vi "Update Methods Event Unbundlers.vi"(8 "error in (no error)":errorcluster, 10 "RPC Method Parameters":T1, 11 "LVClassLibrary in":refnum<vi>) -> (0 "error out":errorcluster, 3 "LVClassLibrary out":refnum<vi>)   [LabVIEW 2019, in "gRPC Template Creation Utility.lvlib"]
uses:
  gRPC Template Creation Utility.lvlib
  TypeDefs/RPC Method Parameters.ctl
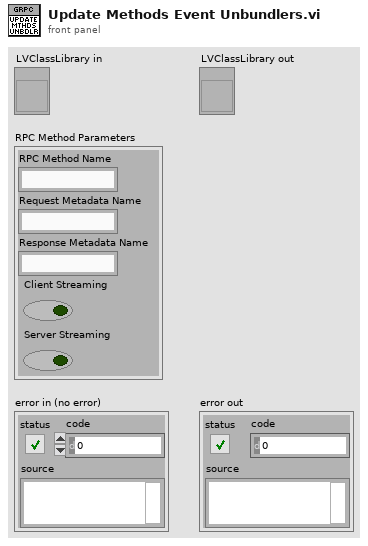
[diagram p1: front panel]
types:
  T1 = typedef "gRPC Template Creation Utility.lvlib/RPC Method Parameters.ctl" = cluster{"RPC Method Name":string, "Request Metadata Name":string, "Response Metadata Name":string, "Client Streaming":bool, "Server Streaming":bool}
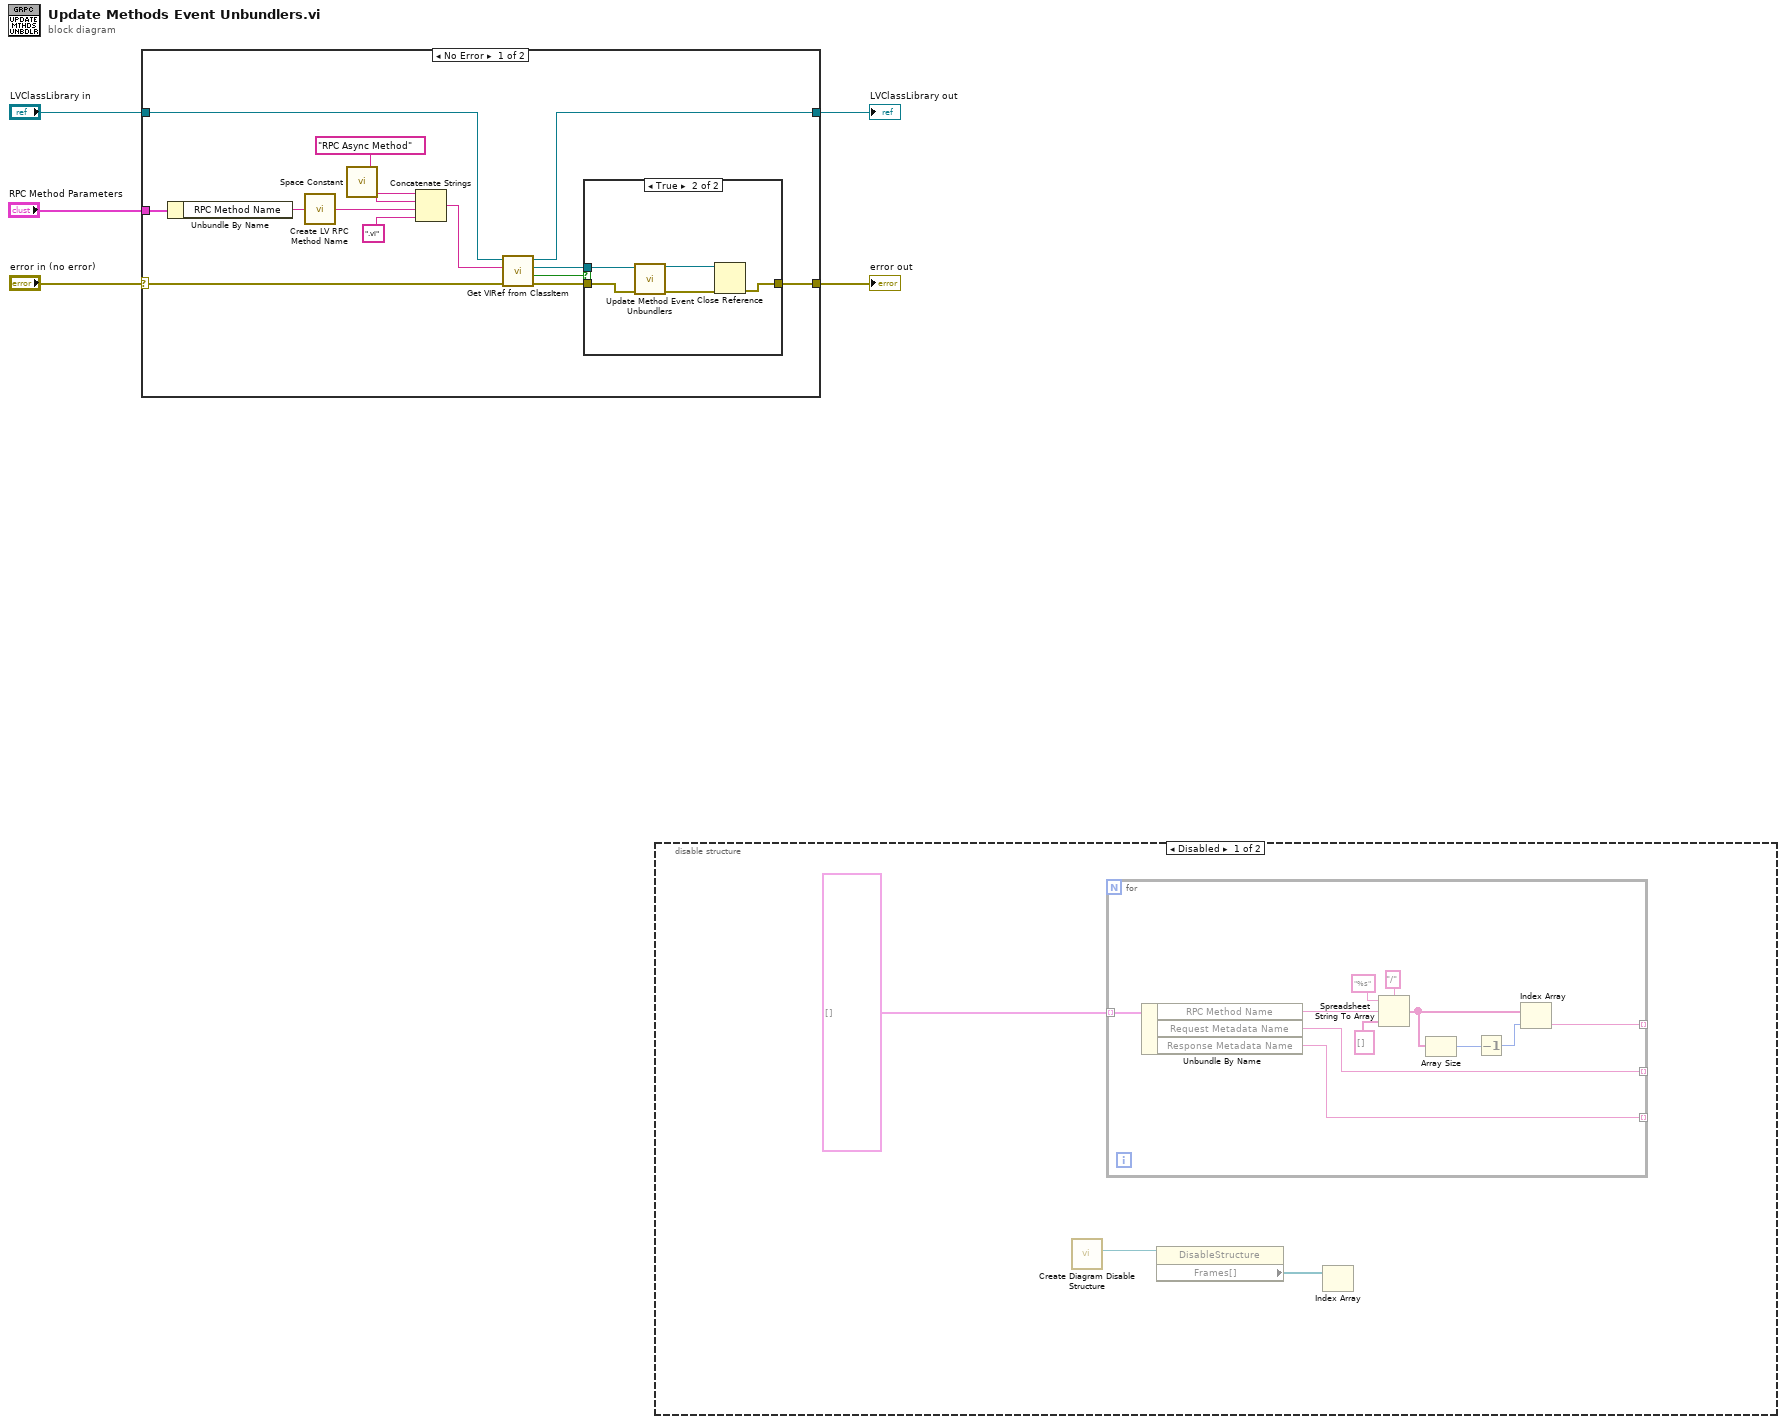
[diagram p0: block diagram]
diagram:
  n1 = case shown="No Error" "error in (no error)" {
    selector: "error in (no error)" -> [w19 w27]
    tunnel: [w10 w26] -> w5
    tunnel: "LVClassLibrary in" -> [w14 w26]
    tunnel: [w9 w27] -> w3
    tunnel: "RPC Method Parameters" -> [w8 _]
    frame No Error {
      n2 = Unbundle By Name(w8) -> ("RPC Method Name"=w7:string)
      n3 = call "Create LV RPC Method Name.vi"("Proto Parser RPC Method Name in"=w7) -> ("LV RPC Method Name out"=w6:string)
      n4 = call <vilib>:"Space Constant.vi"() -> ("String"=w17:string)
      n5 = Concatenate Strings("RPC Async Method" ("regular expression"), w17, w6, ".vi" ("string")) -> (w15:string)
      n6 = call "Get VIRef from ClassItem.vi"("error in (no error)"=w19, "Item Name"=w15, "LVClassLibrary in"=w14) -> ("error out"=w13:errorcluster, "Found ?"=w11:bool, "VIref out"=w12:refnum<vi>, "LVClassLibrary out"=w10:refnum<vi>)  [unwired: 5 in]
      n7 = case shown="True" w11 {
        tunnel: [w20 w25] -> w9
        tunnel: w13 -> [w20 w24]
        tunnel: w12 -> [_ w23]
        frame False {
        }
        frame True {
          n8 = call "Update Method Event Unbundlers.vi"("error in (no error)"=w24, "VI ref in"=w23) -> ("error out"=w22:errorcluster, "VI ref out"=w21:refnum<vi>)  [unwired: 7 in, 1 out]
          n9 = Close Reference(reference=w21, error in (no error)=w22) -> (error out=w25:errorcluster)
        }
      }
    }
    frame Error {
    }
  }
  "error out" <- w3
  "LVClassLibrary out" <- w5
  n10 = disable-structure shown="Disabled" {
    frame Disabled {
      n11 = call "Create Diagram Disable Structure.vi"() -> ("DDS  Ref out"=w28:refnum<vi>)  [unwired: 9 in, 2 out]
      n12 = for {
        tunnel: T1[] [] ("RPC Method Parameters") -> [w41] mode=indexing
        tunnel: [w33] -> _ mode=indexing
        tunnel: [w32] -> _ mode=indexing
        tunnel: [w31] -> _ mode=indexing
        n13 = Unbundle By Name(w41) -> ("RPC Method Name"=w34:string, "Request Metadata Name"=w32:string, "Response Metadata Name"=w31:string)
        n14 = Spreadsheet String To Array(delimiter (Tab)="/", format string="%s", spreadsheet string=w34, array type (2D Dbl)=string[] []) -> (array=w35:string[])
        n15 = Array Size(array=w35) -> (size(s)=w37:i32)
        n16 = Decrement(x=w37) -> (x-1=w36:i32)
        n17 = Index Array(array=w35, index=w36) -> (element=w33:string)
      }
      n18 = property class="DisableStructure"(reference=w28) -> ("Frames[]"=w29:refnum<vi>[])  [unwired: 1 in, 2 out]
      n19 = Index Array(array=w29) -> ()  [unwired: 1 in, 1 out]
    }
    frame Enabled {
    }
  }
